vi "Stopped.vi"(6 "Teller":T1 {"AbsoluteTime" format="%<%x %.3X>T"}, 8 "Error in":errorcluster, 9 "Error":errorcluster, 10 "Actor":refnum<class "Actor.lvclass">, 11 "Base Actor in":refnum<class "BaseActor.lvclass">) -> (0 "Error out":errorcluster, 3 "Base Actor out":refnum<class "BaseActor.lvclass">)   [LabVIEW 2020, in "jettl.lvlib" / "BaseActor.lvlib" / "BaseActor.lvclass"]
uses:
  BaseActor.lvclass
  BaseActor.lvclass/BaseActor.ctl
  jettl.lvlib
  Lifetime.ctl
  Actor/Actor.lvclass
  MessageMetadata.ctl
  TellOrigin.ctl
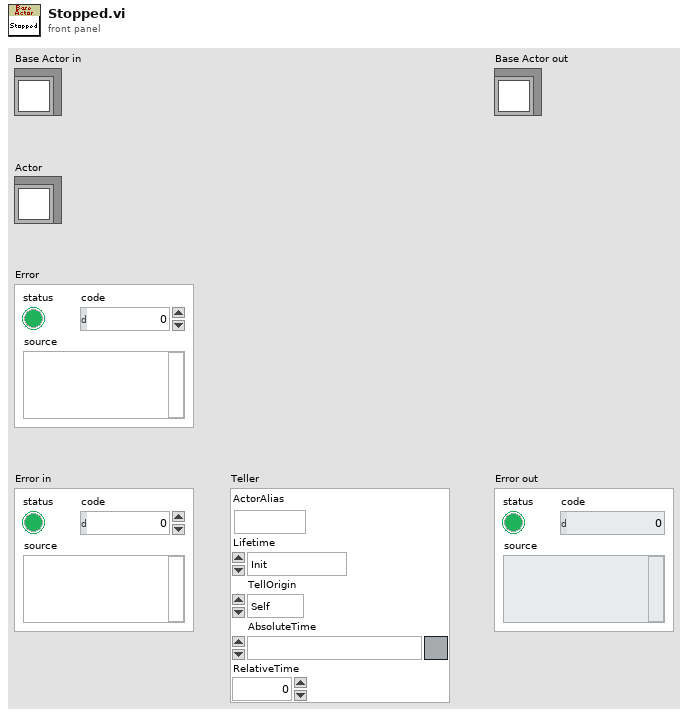
[diagram p1: front panel]
types:
  T1 = typedef "jettl.lvlib/MessageMetadata.ctl" = cluster{"ActorAlias":string, "Lifetime":T2, "TellOrigin":T3, "AbsoluteTime":timestamp, "RelativeTime":dbl}
  T2 = typedef "jettl.lvlib/Lifetime.ctl" = enum16{"Init", "Spawn", "Setup", "TeardownBeforeRunning", "Running", "StopCalled", "StoppingWithComponents", "StoppingNoComponents", "TeardownAfterRunning", "Stopped"}
  T3 = typedef "jettl.lvlib/TellOrigin.ctl" = enum16{"Self", "Mediator", "Component"}
  T4 = typedef "jettl.lvlib/ComponentActorMap.ctl" = map{string, T5}
  T5 = typedef "jettl.lvlib/Actor.ctl" = cluster{"Messages":T6, "ActorAlias":string, "ActorType":T9, "Transport":refnum<user-event>, "VIRef":refnum<vi>}
  T6 = typedef "jettl.lvlib/Messages.ctl" = cluster{"Listen":T7, "TellSelf":T7, "TellMediator":T7, "TellComponentMap":T8}
  T7 = typedef "jettl.lvlib/MessageSet.ctl" = set{refnum<class "Message.lvclass">}
  T8 = typedef "jettl.lvlib/TellComponentMap.ctl" = map{string, T7}
  T9 = typedef "jettl.lvlib/ActorType.ctl" = enum16{"Mediator", "Component"}
  T10 = typedef "jettl.lvlib/Lifetime.ctl" = enum16{"Init", "Spawn", "Setup", "Teardown Before Running", "Running", "Stop Called", "Stopping With Children", "Stopping Without Children", "Teardown After Running", "Stopped"}
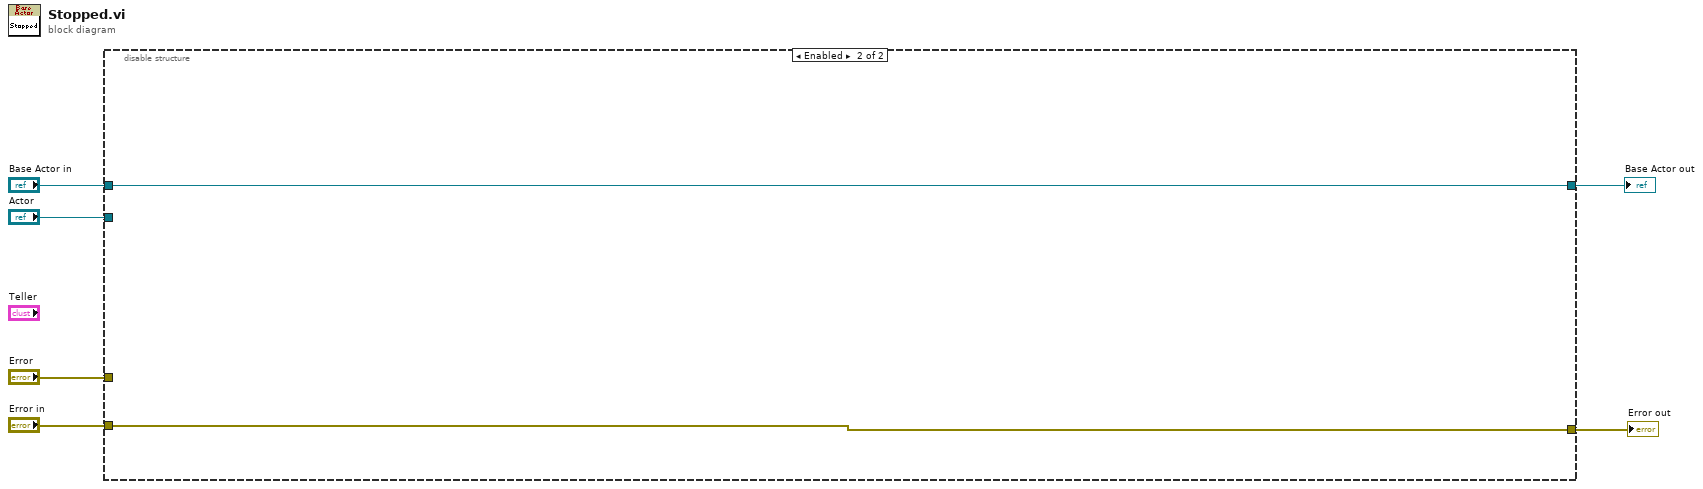
[diagram p0: block diagram]
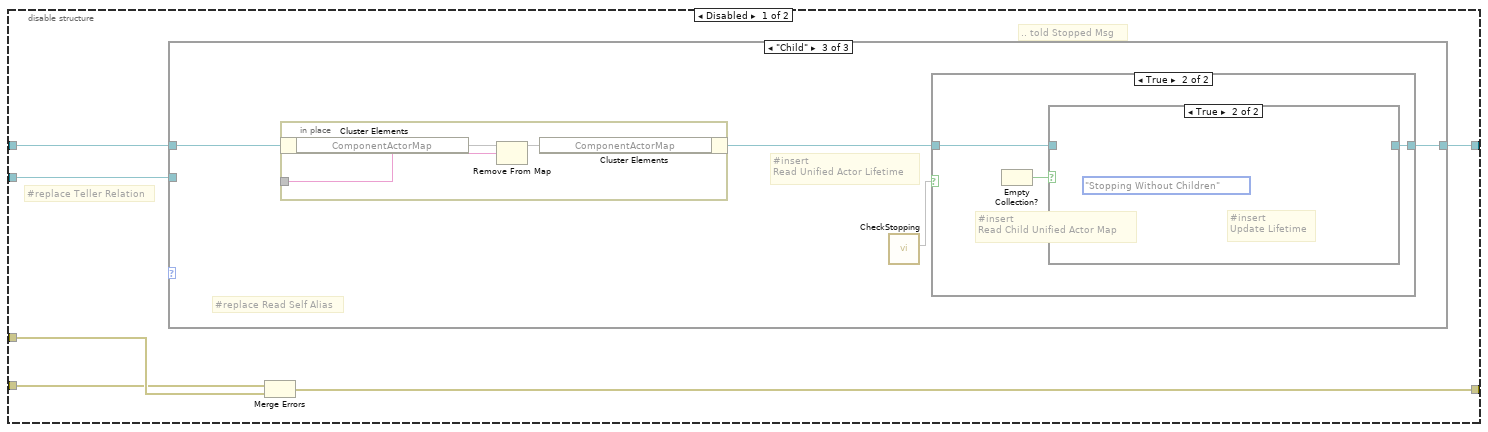
[diagram p2: hidden frame]
diagram:
  n1 = disable-structure shown="Enabled" {
    disable-tunnel: [w12 w31] -> w6
    disable-tunnel: "Base Actor in" -> [w11 w31]
    disable-tunnel: "Actor" -> [w10 _]
    disable-tunnel: "Error" -> [w9 _]
    disable-tunnel: "Error in" -> [w8 w32]
    disable-tunnel: [w7 w32] -> w1
    frame Disabled {
      # "#replace Teller Relation"
      # ".. told Stopped Msg"
      n2 = case shown="\"Child\"" {
        selector: _ -> [_ _ _]
        tunnel: w11 -> [w13 w14 w16]
        tunnel: [w13 w14 w18] -> w12
        tunnel: w10 -> [_ _ w17]
        frame "Self" {
          # "Case will not fundamentally execute"
        }
        frame "Parent" {
          # "Case will not fundamentally execute"
        }
        frame "Child" {
          # "#insert\nRead Unified Actor Lifetime"
          # "#replace Read Self Alias"
          n3 = in-place {
            in-place-border: [w22] -> _
            n4 = in-place-cluster #1(w16) -> ("ComponentActorMap"=w21:T4)
            n5 = Remove From Map(11:w21) -> (3:w20:T4, 10:w22:string)  [unwired: 2 out]
            n6 = in-place-cluster #1("ComponentActorMap"=w20) -> (w15:refnum<class "BaseActor.lvclass">)
          }
          n7 = call "CheckStopping.vi"() -> (2:w19)  [unwired: 10 in, 1 out]
          n8 = case shown="True" w19 {
            tunnel: w15 -> [w23 w24]
            tunnel: [w23 w26] -> w18
            frame False {
            }
            frame True {
              # "#insert\nRead Child Unified Actor Map"
              n9 = Empty Collection?() -> (0:w25:bool)  [unwired: 1 in]
              n10 = case shown="True" w25 {
                tunnel: [w27 w28] -> w26
                tunnel: w24 -> [w27 w29]
                frame False {
                }
                frame True {
                  w30 = Lifetime."Stopping Without Children" ("Lifetime")
                  # "#insert\nUpdate Lifetime"
                }
              }
            }
          }
        }
      }
      n11 = Merge Errors(w8, w9) -> (w7:errorcluster)
    }
    frame Enabled {
    }
  }
  "Base Actor out" <- w6
  "Error out" <- w1
